vi "GetVisPaths.vi"(8 "ErrorArray in":errorcluster[](array[cluster]), 10 "PathsToVisApps":string[](array[string])) -> (0 "ErrorArray out":errorcluster[](array[cluster]), 2 "VisPaths":path[](array[path]))   [LabVIEW 2014, in "Visualization.lvlib"]
uses:
  Visualization.lvlib
  <userlib>/NIST/NISTErrorLib/NISTErrorLib.lvlib
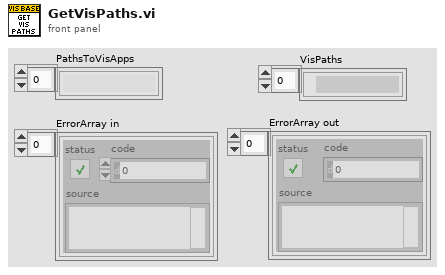
[diagram p1: front panel]
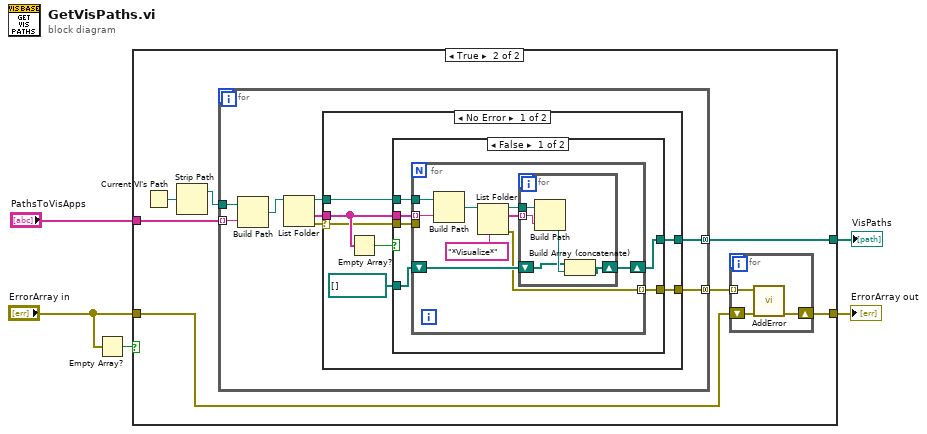
[diagram p0: block diagram]
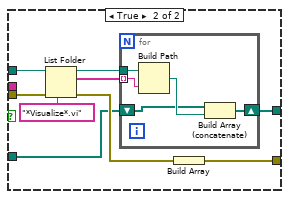
[diagram p3: hidden frame]
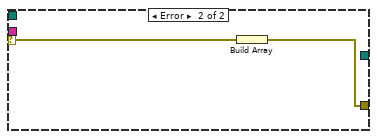
[diagram p4: hidden frame]
diagram:
  n1 = Empty Array?(array="ErrorArray in") -> (empty?=w3:bool)
  n2 = case shown="True" w3 {
    tunnel: "ErrorArray in" -> [w6 w9]
    tunnel: "PathsToVisApps" -> [_ w13]
    tunnel: [w6 w8] -> w5
    tunnel: [_ w7] -> w1
    frame False {
    }
    frame True {
      n3 = Current VI's Path() -> (path=w12:path)
      n4 = Strip Path(path=w12) -> (stripped path=w11:path)  [unwired: 1 out]
      n5 = for {
        tunnel: w13 -> [w24] mode=indexing
        tunnel: w11 -> [w23]
        tunnel: [w18] -> w7 mode=concatenating
        tunnel: [w17] -> w10 mode=concatenating
        n6 = Build Path(base path=w23, name or relative path=w24) -> (appended path=w22:path)
        n7 = List Folder(path=w22) -> (path out=w20:path, folder names=w19:string[], error out=w21:errorcluster)  [unwired: 3 in, 1 out]
        n8 = case shown="No Error" w21 {
          selector: w21 -> [w29 w67]
          tunnel: w20 -> [w28 _]
          tunnel: w19 -> [w30 _]
          tunnel: [w27 _] -> w18
          tunnel: [w26 w66] -> w17
          frame No Error {
            n9 = Empty Array?(array=w30) -> (empty?=w31:bool)
            n10 = case shown="False" w31 {
              tunnel: w30 -> [w37 _]
              tunnel: w29 -> [w36 w59]
              tunnel: w28 -> [w35 w60]
              tunnel: [w34 w55] -> w27
              tunnel: [w32 w52] -> w26
              tunnel: path[] [] -> [w33 w53]
              frame False {
                n11 = for {
                  tunnel: w37 -> [w46] mode=indexing
                  tunnel: w36 -> [_]
                  tunnel: w35 -> [w45]
                  shift-right: [w39] -> w34
                  shift-left: w33 -> [w40]
                  tunnel: [w38] -> w32 mode=indexing
                  n12 = Build Path(base path=w45, name or relative path=w46) -> (appended path=w44:path)
                  n13 = List Folder(path=w44, pattern="*Visualize*") -> (path out=w42:path, filenames=w41:string[], error out=w38:errorcluster)  [unwired: 2 in, 1 out]
                  n14 = for {
                    tunnel: w42 -> [w51]
                    tunnel: w41 -> [w50] mode=indexing
                    shift-right: [w47] -> w39
                    shift-left: w40 -> [w48]
                    n15 = Build Path(base path=w51, name or relative path=w50) -> (appended path=w49:path)
                    n16 = Build Array (concatenate)(w48, w49) -> (w47:path[])
                  }
                }
              }
              frame True {
                n17 = List Folder(path=w60, pattern="*Visualize*.vi", error in=w59) -> (path out=w57:path, filenames=w56:string[], error out=w54:errorcluster)  [unwired: 1 in, 1 out]
                n18 = for {
                  tunnel: w57 -> [w65]
                  tunnel: w56 -> [w64] mode=indexing
                  shift-right: [w62] -> w55
                  shift-left: w53 -> [w61]
                  n19 = Build Path(base path=w65, name or relative path=w64) -> (appended path=w63:path)
                  n20 = Build Array (concatenate)(w61, w63) -> (w62:path[])
                }
                n21 = Build Array(w54) -> (w52:errorcluster[])
              }
            }
          }
          frame Error {
            n22 = Build Array(w67) -> (w66:errorcluster[])
          }
        }
      }
      n23 = for {
        tunnel: w10 -> [w16] mode=indexing
        shift-right: [w14] -> w8
        shift-left: w9 -> [w15]
        n24 = call <userlib>:"AddError.vi"("ErrorArray"=w15, "error in (no error)"=w16) -> ("ErrorArray"=w14:errorcluster[])  [unwired: 8 in, 1 out]
      }
    }
  }
  "ErrorArray out" <- w5
  "VisPaths" <- w1
